vi "ActBalance.vi"(10 "MaxSpeed (ft/s)":dbl) -> (1 "XSpeedDemand":dbl, 3 "Done":bool)   [LabVIEW 2023]
doc: "Robot begins balancing towards the \"GyroZero\" position. \n\nInputs:\n-- MaxSpeed -- Double -- in ft/s, the MaxSpeed the robot can go (Has no effect above 1.5)\n\n\nOutputs:\n-- Done -- Bool -- has the robot reached its target distance\n-- LeftSpeedDemand -- Double -- Speed Demand for left drive train inorder to reach target -- \n-- RightSpeedDemand -- Double -- Speed Demand for left drive train inorder to reach target --"
uses:
  <vilib>/Rock Robotics/WPI/ThirdParty/JAS_Junk/TrajLib/VI/Util_GetTime_U32.vi
  <vilib>/Rock Robotics/WPI/ThirdParty/JAS_Junk/TrajLib/LinearFilter_ResetToValue.vi
  <vilib>/Rock Robotics/WPI/ThirdParty/JAS_Junk/TrajLib/LinearFilter_Calculate.vi
  <vilib>/Rock Robotics/WPI/ThirdParty/JAS_Junk/TrajLib/Timer_New.vi
  <vilib>/Rock Robotics/SystemInterfaces/Utilities/FPGA_UtilitiesRead LocalTime.vi
  <vilib>/Rock Robotics/WPI/ThirdParty/JAS_Junk/TrajLib/VI/Util_GetTime_U64.vi
  <vilib>/Rock Robotics/Network Tables/NT Write Number.vi
  <vilib>/Rock Robotics/WPI/ThirdParty/JAS_Junk/TrajLib/LinearFilter_MovingAverage.vi
  <vilib>/Rock Robotics/WPI/ThirdParty/JAS_Junk/TrajLib/LinearFilter_LowPassBW1.vi
  <vilib>/Rock Robotics/WPI/ThirdParty/JAS_Junk/TrajLib/LinearFilter_LowPassBW2.vi
  <vilib>/Rock Robotics/WPI/ThirdParty/JAS_Junk/TrajLib/LinearFilter_HighPassBW1.vi
  <vilib>/Rock Robotics/WPI/ThirdParty/JAS_Junk/TrajLib/LinearFilter_HighPassBW2.vi
  <vilib>/Utility/semaphor.llb/Obtain Semaphore Reference.vi
  <vilib>/Rock Robotics/WPI/ThirdParty/JAS_Junk/TrajLib/Timer_Reset.vi
  <vilib>/Rock Robotics/WPI/ThirdParty/JAS_Junk/TrajLib/Timer_Start.vi
  <vilib>/Rock Robotics/WPI/ThirdParty/JAS_Junk/TrajLib/Timer_HasPeriodPassedOnce.vi
  <vilib>/Rock Robotics/WPI/ThirdParty/JAS_Junk/TrajLib/Timer_Stop.vi
  <vilib>/Rock Robotics/WPI/ThirdParty/JAS_Junk/TrajLib/Trajectory_Library.lvlib
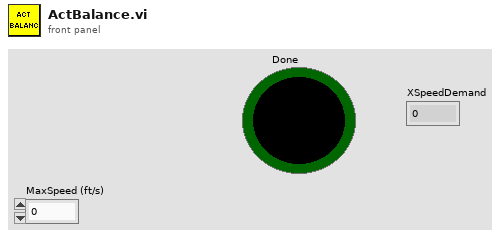
[diagram p1: front panel]
types:
  T1 = enum16{"Moving Average", "Low Pass 1st Order Butterworth", "Low Pass 2nd Order Butterworth", "High Pass 1st Order Butterworth", "High Pass 2nd Order Butterworth"}
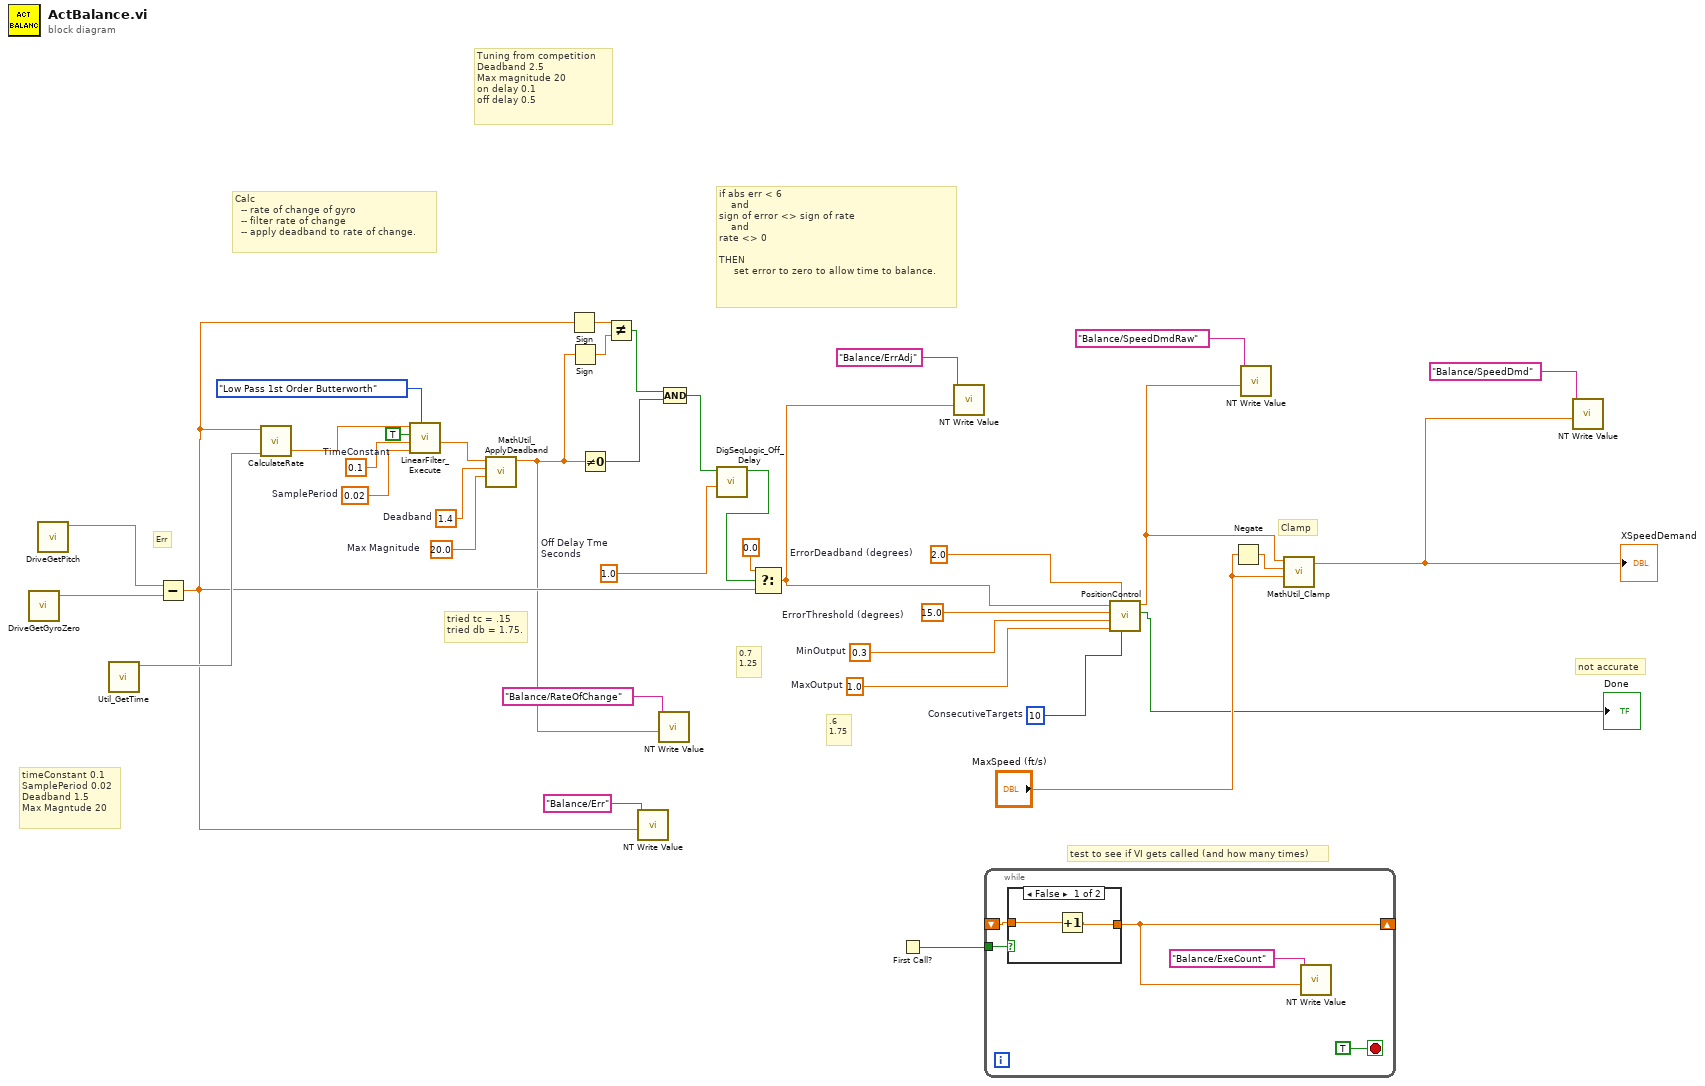
[diagram p0: block diagram]
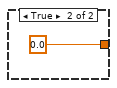
[diagram p2: hidden frame]
diagram:
  w3 = 1.0  # Off Delay Tme Seconds
  w22 = 0.02  # SamplePeriod
  w21 = 0.1  # TimeConstant
  w23 = 20.0  # Max Magnitude
  w24 = 1.4  # Deadband
  w33 = 1.0  # MaxOutput
  w34 = 0.3  # MinOutput
  w32 = 10  # ConsecutiveTargets
  w37 = 2.0  # ErrorDeadband (degrees)
  w38 = 15.0  # ErrorThreshold (degrees)
  # "Tuning from competition\nDeadband 2.5\nMax magnitude 20\non delay 0.1\noff delay 0.5"
  # ".6\n1.75"
  # "test to see if VI gets called (and how many times)"
  # "not accurate"
  # "if abs err < 6 \n    and\nsign of error <> sign of rate\n    and\nrate <> 0\n\nTHEN\n     set error to zero to allow time to balance."
  # "tried tc = .15\ntried db = 1.75."
  # "Calc\n  -- rate of change of gyro\n  -- filter rate of change\n  -- apply deadband to rate of change."
  # "Err"
  # "0.7\n1.25"
  # "timeConstant 0.1\nSamplePeriod 0.02\nDeadband 1.5\nMax Magntude 20"
  # "Clamp"
  n1 = call "DriveGetGyroZero.vi"() -> ("GyroZero"=w31:dbl)  [unwired: 11 in]
  n2 = call "DriveGetPitch.vi"() -> ("Pitch"=w30:dbl)  [unwired: 11 in]
  n3 = call <vilib>:"Util_GetTime.vi"() -> ("FPGA_Time_Seconds"=w25:dbl)  [unwired: 9 in, 2 out]
  n4 = Subtract(x=w30, y=w31) -> (x-y=w14:dbl)
  n5 = call "CalculateRate.vi"("Time (s)"=w25, "Distance (units)"=w14) -> ("Rate (units/s)"=w17:dbl)  [unwired: 9 in]
  n6 = call <vilib>:"LinearFilter_Execute.vi"("Filter Type"=T1."Low Pass 1st Order Butterworth", "SamplePeriod"=w22, "TimeConstant"=w21, "Enable"=TRUE, "Input"=w17) -> ("Output"=w16:dbl)  [unwired: 5 in, 1 out]
  n7 = call <vilib>:"MathUtil_ApplyDeadband.vi"("Max Magnitude"=w23, "Deadband"=w24, "Value"=w16) -> ("Result"=w5:dbl)  [unwired: 8 in]
  n8 = Sign(1:w14) -> (0:w28:dbl)
  n9 = Sign(1:w5) -> (0:w27:dbl)
  n10 = Not Equal To 0?(x=w5) -> (x != 0?=w18:bool)
  n11 = Not Equal?(x=w28, y=w27) -> (x != y?=w26:bool)
  n12 = call-poly <vilib>:"NT Write Value.vi"("value"=w14, "name"="Balance/Err") -> ()  [unwired: 9 in, 1 out]
  n13 = call-poly <vilib>:"NT Write Value.vi"("value"=w5, "name"="Balance/RateOfChange") -> ()  [unwired: 9 in, 1 out]
  n14 = Compound Arithmetic op=AND(w26, w18) -> (w1:bool)
  n15 = call <vilib>:"DigSeqLogic_Off_Delay.vi"("Delay"=w3, "Input"=w1) -> ("Output"=w2:bool)  [unwired: 8 in, 1 out]
  n16 = Select(t=0.0, s=w2, f=w14) -> (s? t:f=w12:dbl)
  n17 = First Call?() -> (First Call?: T/F=w7:bool)
  n18 = call-poly <vilib>:"NT Write Value.vi"("value"=w12, "name"="Balance/ErrAdj") -> ()  [unwired: 9 in, 1 out]
  n19 = while {
    tunnel: w7 -> [w42]
    shift-right: [w39] -> _
    shift-left: _ -> [w41]
    stop <- TRUE stop-if-true
    n20 = case shown="False" w42 {
      tunnel: [w45 0.0] -> w39
      tunnel: w41 -> [w44 _]
      frame False {
        n21 = Increment(x=w44) -> (x+1=w45:dbl)
      }
      frame True {
      }
    }
    n22 = call-poly <vilib>:"NT Write Value.vi"("value"=w39, "name"="Balance/ExeCount") -> ()  [unwired: 9 in, 1 out]
  }
  n23 = call "PositionControl.vi"("ConsecutiveTargets"=w32, "ErrorDeadband"=w37, "MaxOutput"=w33, "MinOutput"=w34, "ErrorThreshold"=w38, "Error"=w12) -> ("OnTarget"=→"Done":bool, "OutputValue"=w10:dbl)  [unwired: 3 in, 1 out]
  n24 = Negate(x="MaxSpeed (ft/s)") -> (-x=w36:dbl)
  n25 = call-poly <vilib>:"NT Write Value.vi"("value"=w10, "name"="Balance/SpeedDmdRaw") -> ()  [unwired: 9 in, 1 out]
  n26 = call <vilib>:"MathUtil_Clamp.vi"("High Limit"="MaxSpeed (ft/s)", "Low Limit"=w36, "Value"=w10) -> ("Result"=w8:dbl)  [unwired: 8 in]
  "XSpeedDemand" <- w8
  n27 = call-poly <vilib>:"NT Write Value.vi"("value"=w8, "name"="Balance/SpeedDmd") -> ()  [unwired: 9 in, 1 out]
